vi "Recorder inquiry.vi"(7 "Channel  (1: CH1)":u16(ring)=1 items=["CH1"=1, "CH2"=2, "CH3"=3, "CH4"=4], 8 "error in (no error)":errorcluster, 11 "VISA resource name":refnum<visa-resource-name>) -> (0 "error out":errorcluster, 1 "Groups":dbl, 2 "Period":dbl, 3 "VISA resource name out":refnum<visa-resource-name>, 4 "Memory Path":string)   [LabVIEW 2020, in "GPP.lvlib"]
uses:
  GPP.lvlib
  Function/VISA_COMMON.ctl
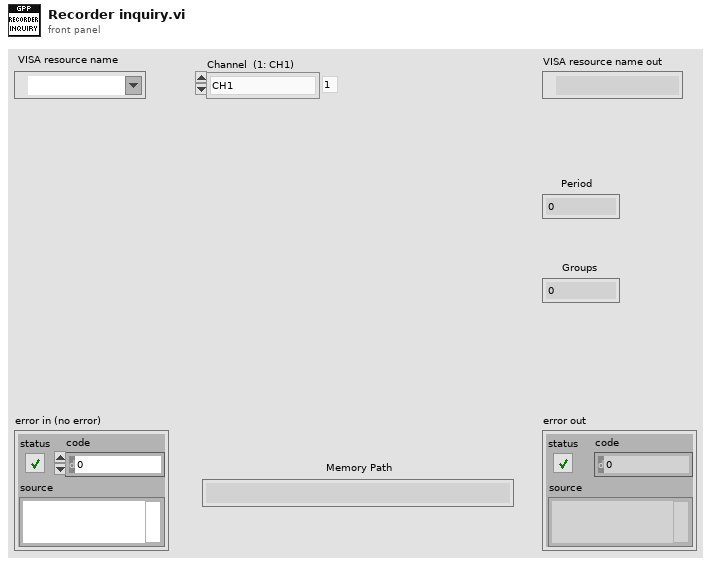
[diagram p1: front panel]
types:
  T1 = typedef "GPP.lvlib/VISA_COMMON.ctl" = enum16{"Initial", "Write CMD", "Read Result", "Read History", "Close"}
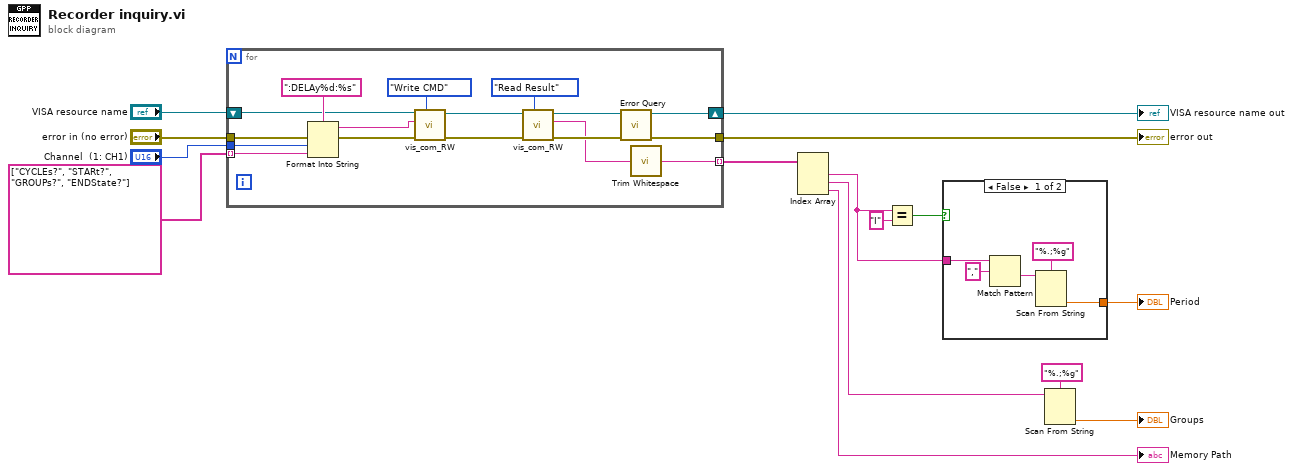
[diagram p0: block diagram]
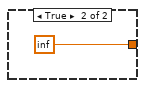
[diagram p2: hidden frame]
diagram:
  n1 = for {
    tunnel: "error in (no error)" -> [w26]
    tunnel: "Channel  (1: CH1)" -> [w24]
    tunnel: string[] ["CYCLEs?", "STARt?", "GROUPs?", "ENDState?"] -> [w21] mode=indexing
    tunnel: [w22] -> w8
    tunnel: [w18] -> w12 mode=indexing
    shift-right: [w16] -> w7
    shift-left: "VISA resource name" -> [w20]
    n2 = Format Into String(format string=":DELAy%d:%s", error in=w26, w24, w21) -> (resulting string=w19:string, error out=w25:errorcluster)  [unwired: 1 in]
    n3 = call "vis_com_RW.vi"("Funciton"=VISA_COMMON."Write CMD", "error in (no error)"=w25, "CMD String"=w19, "VISA resource in"=w20) -> ("error out"=w30:errorcluster, "VISA resource out"=w29:refnum<visa-resource-name>)  [unwired: 5 in, 1 out]
    n4 = call "vis_com_RW.vi"("Funciton"=VISA_COMMON."Read Result", "error in (no error)"=w30, "VISA resource in"=w29) -> ("error out"=w27:errorcluster, "Result"=w17:string, "VISA resource out"=w28:refnum<visa-resource-name>)  [unwired: 6 in]
    n5 = call "Error Query.vi"("error in (no error)"=w27, "VISA resource name"=w28) -> ("error out"=w22:errorcluster, "VISA resource name out"=w16:refnum<visa-resource-name>)  [unwired: 6 in, 2 out]
    n6 = call <vilib>:"Trim Whitespace.vi"("string"=w17) -> ("trimmed string"=w18:string)  [unwired: 1 in]
  }
  "error out" <- w8
  "VISA resource name out" <- w7
  n7 = Index Array(array=w12) -> (element #1=w1:string, element #2=w10:string, element #3=→"Memory Path":string)  [unwired: 3 in]
  n8 = Equal?(x=w1, y="I") -> (x = y?=w3:bool)
  n9 = case shown="False" w3 {
    tunnel: [w34 inf ("t")] -> w2
    tunnel: w1 -> [w33 _]
    frame False {
      n10 = Match Pattern(string=w33, regular expression=",") -> (after substring=w35:string)  [unwired: 1 in, 3 out]
      n11 = Scan From String(format string="%.;%g", input string=w35) -> (output 1=w34:dbl)  [unwired: 3 in, 3 out]
    }
    frame True {
    }
  }
  "Period" <- w2
  n12 = Scan From String(format string="%.;%g", input string=w10) -> (output 1=→"Groups":dbl)  [unwired: 3 in, 3 out]
